vi "Write All Variables.vi"(8 "error in (no error)":errorcluster, 10 "Correct. vars.":T1, 11 "Correct params in":refnum<class "CV-Correction.lvclass">) -> (0 "error out":errorcluster, 3 "Correct params out":refnum<class "CV-Correction.lvclass">)   [LabVIEW 2013, in "CameraVision.lvlib" / "CV-Correction.lvclass"]
uses:
  CV-Correction.lvclass
  Correction-variables.ctl
  CV-Correction.lvclass/CV-Correction.ctl
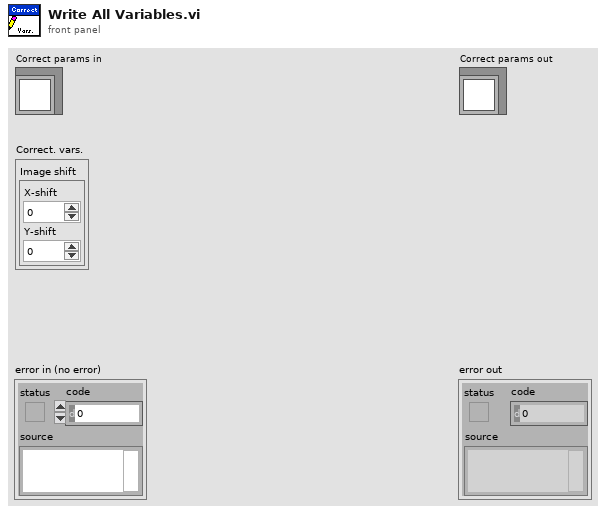
[diagram p1: front panel]
types:
  T1 = typedef "CameraVision.lvlib/CV-Correction.lvclass/Correction-variables.ctl" = cluster{"Image shift":cluster{"X-shift":i32, "Y-shift":i32}}
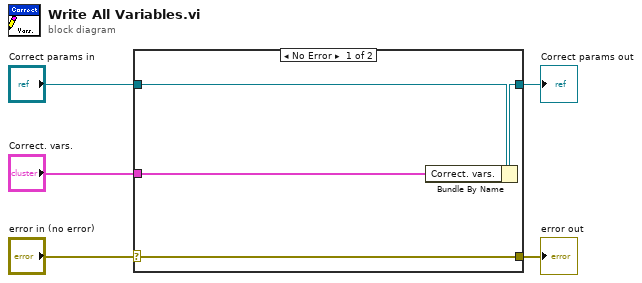
[diagram p0: block diagram]
diagram:
  n1 = case shown="No Error" "error in (no error)" {
    selector: "error in (no error)" -> [w9 w10]
    tunnel: [w9 w10] -> w4
    tunnel: [w7 w11] -> w2
    tunnel: "Correct params in" -> [w8 w11]
    tunnel: "Correct. vars." -> [w6 _]
    frame No Error {
      n2 = Bundle By Name(cluster=w8, "Correct. vars."=w6) -> (w7:refnum<class "CV-Correction.lvclass">)
    }
    frame Error {
    }
  }
  "error out" <- w4
  "Correct params out" <- w2
